vi "subVI QCam Grab Frame.vi"(3 "error in":errorcluster, 4 "Image Pointer In":T1, 5 "cameraId":u32) -> (0 "error out":errorcluster, 1 "Image Pointer Out":T1, 2 "cameraId out":u32)   [LabVIEW 2012]
uses:
  <vilib>/vision/Image Controls.llb/IMAQ Image.ctl
  SubVI/ProSCI Global.vi
  SubVI/ProSCI DebugGlobal.vi
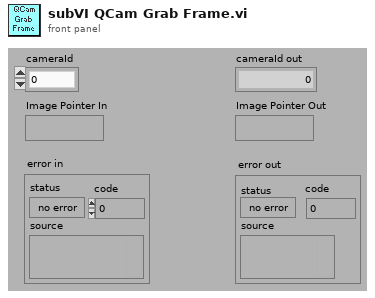
[diagram p1: front panel]
types:
  T1 = typedef "IMAQ Image.ctl" = refnum<image>
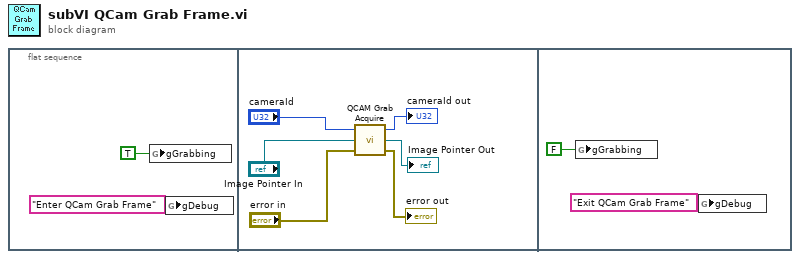
[diagram p0: block diagram]
diagram:
  n1 = flat-sequence {
    frame #0 {
      n2 = global write "ProSCI Global.vi" "gGrabbing"(TRUE ("gGrabbing")) -> ()
      n3 = global write "ProSCI DebugGlobal.vi" "gDebug"("Enter QCam Grab Frame" ("gDebug")) -> ()
    }
    frame #1 {
      n4 = call "QCAM Grab Acquire.vi"("error in (no error)"="error in", "Image"="Image Pointer In", "cameraId"="cameraId") -> ("error out"=→"error out":errorcluster, "Image Out"=→"Image Pointer Out":T1, "cameraId out"=→"cameraId out":u32)
    }
    frame #2 {
      n5 = global write "ProSCI Global.vi" "gGrabbing"(FALSE ("gGrabbing")) -> ()
      n6 = global write "ProSCI DebugGlobal.vi" "gDebug"("Exit QCam Grab Frame" ("gDebug")) -> ()
    }
  }
